vi "Color Sensor V3 Add Color Match.vi"(10 "Color":cluster{"R":dbl, "G":dbl, "B":dbl}, 11 "Name":string) -> ()   [LabVIEW 2019]
uses:
  TypeDef/Color Sensor V3 Color Match.ctl
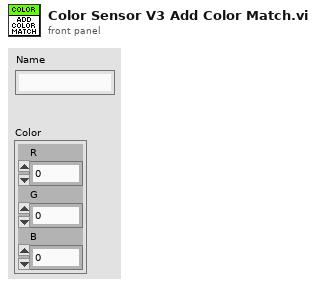
[diagram p1: front panel]
types:
  T1 = typedef "Color Sensor V3 Color Match.ctl" = cluster{"Name":string, "Normalized Color":cluster{"R":dbl, "G":dbl, "B":dbl}}
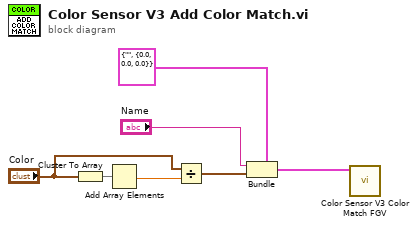
[diagram p0: block diagram]
diagram:
  n1 = Cluster To Array(cluster="Color") -> (array=w4:dbl[])
  n2 = Add Array Elements(numeric array=w4) -> (sum=w3:dbl)
  n3 = Divide(x="Color", y=w3) -> (x/y=w1:cluster{"R":dbl, "G":dbl, "B":dbl})
  n4 = Bundle(cluster=T1 {"Name"="", "Normalized Color"={"R"=0.0, "G"=0.0, "B"=0.0}} ("output cluster"), "Name"="Name", "Normalized Color"=w1) -> (w5:T1)
  n5 = call "Color Sensor V3 Color Match FGV.vi"("Color Match"=w5) -> ()  [unwired: 10 in, 1 out]
